vi "LIN Send Single Message.vi"(0 "NAD":u8 format="%.0x", 1 "LIN Device":T1={"Master Frame(3C)"="MasterReq\nSPA3414_ConfigurationsCMAGeely_CEMCALYPSOSDB34XX0Cfg_LIN3_190709_", "Slave Frame(3D)"="SlaveResp\nSPA3414_ConfigurationsCMAGeely_CEMCALYPSOSDB34XX0Cfg_LIN3_190709_", "Request Schedule"="CEMLIN3DiagRequestSchedule\nSPA3414_ConfigurationsCMAGeely_CEMCALYPSOSDB34XX0Cfg_LIN3_190709_", "Response Schedule"="CEMLIN3DiagResponseSchedule\nSPA3414_ConfigurationsCMAGeely_CEMCALYPSOSDB34XX0Cfg_LIN3_190709_", "Frame Write SCU"="", "Frame Read SCU"="", "LIN Name"=""}, 5 "Msg Wait T":u32=3000, 7 "Retries":i32, 9 "FrameCount":i32=1, 11 "error in (no error)":errorcluster, 12 "Need REQ":bool=TRUE, 13 "Tx Msg":u8[][](array[numeric]) format="%.0x") -> (3 "size":i32, 4 "Rx Msg":u8[](array[numeric]) format="%.0x", 6 "TxRx Data":string[][](array[string]), 8 "Response Good?":bool, 10 "spreadsheet String":string, 15 "error OUT":errorcluster caption="error in (no error)")   [LabVIEW 2018]
uses:
  LIN Device.ctl
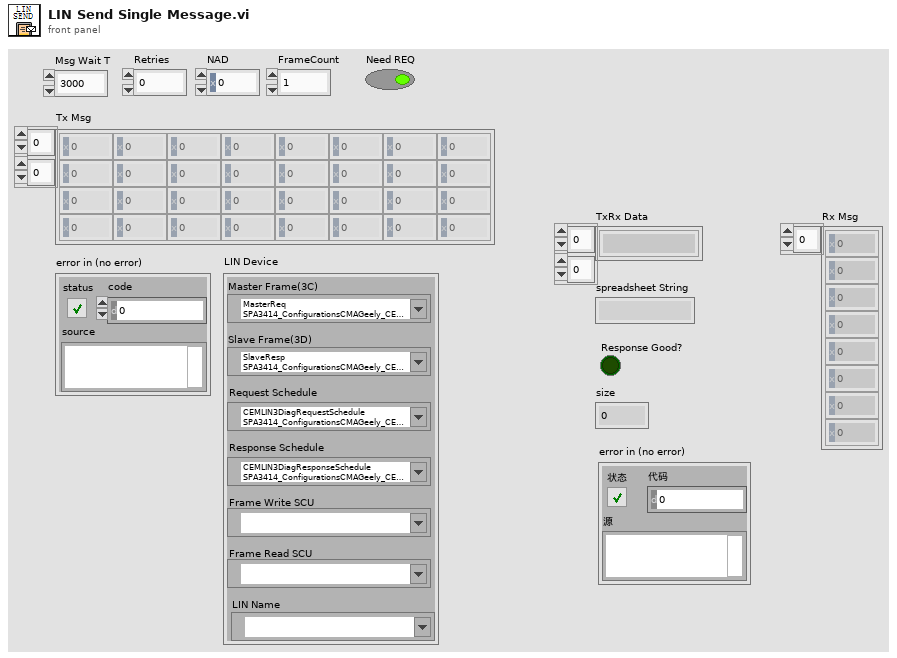
[diagram p1: front panel]
types:
  T1 = typedef "LIN Device.ctl" = cluster{"Master Frame(3C)":refnum<k21>, "Slave Frame(3D)":refnum<k21>, "Request Schedule":refnum<k21>, "Response Schedule":refnum<k21>, "Frame Write SCU":refnum<k21>, "Frame Read SCU":refnum<k21>, "LIN Name":refnum<k21>}
  T2 = cluster{"Tx Msg":u8[][], "NAD":u8, "Retry Counter":i32, "Rx Msg":u8[], "FrameCount":i32, "FF":u8[], "Response Good?":bool, "TxRx Data":string[][], "Message Start Timer":u32, "LIN Device":T1, "element":string[]}
  T3 = typedef "XNET Frame LIN.ctl" = cluster{"timestamp":timestamp, "payload":u8[], "identifier":u32, "type":T4, "event ID":u8, "event slot?":bool, "echo?":bool}
  T4 = typedef "XNET Frame Type LIN.ctl" = u8
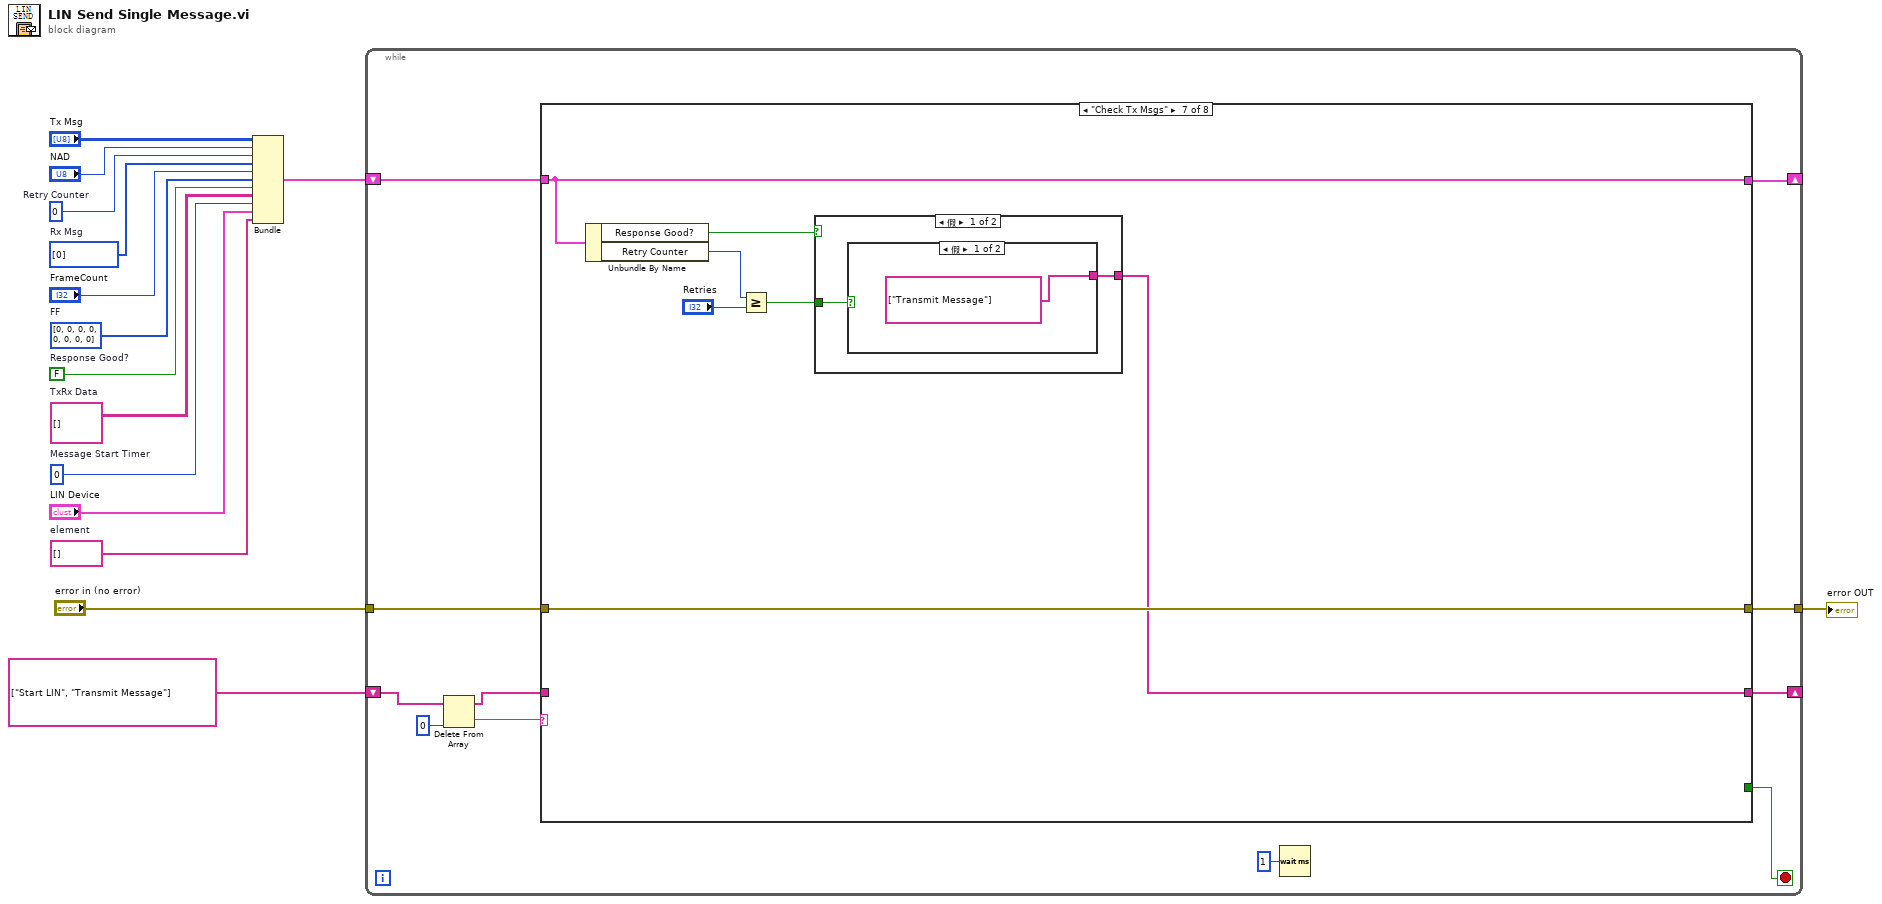
[diagram p0: block diagram]
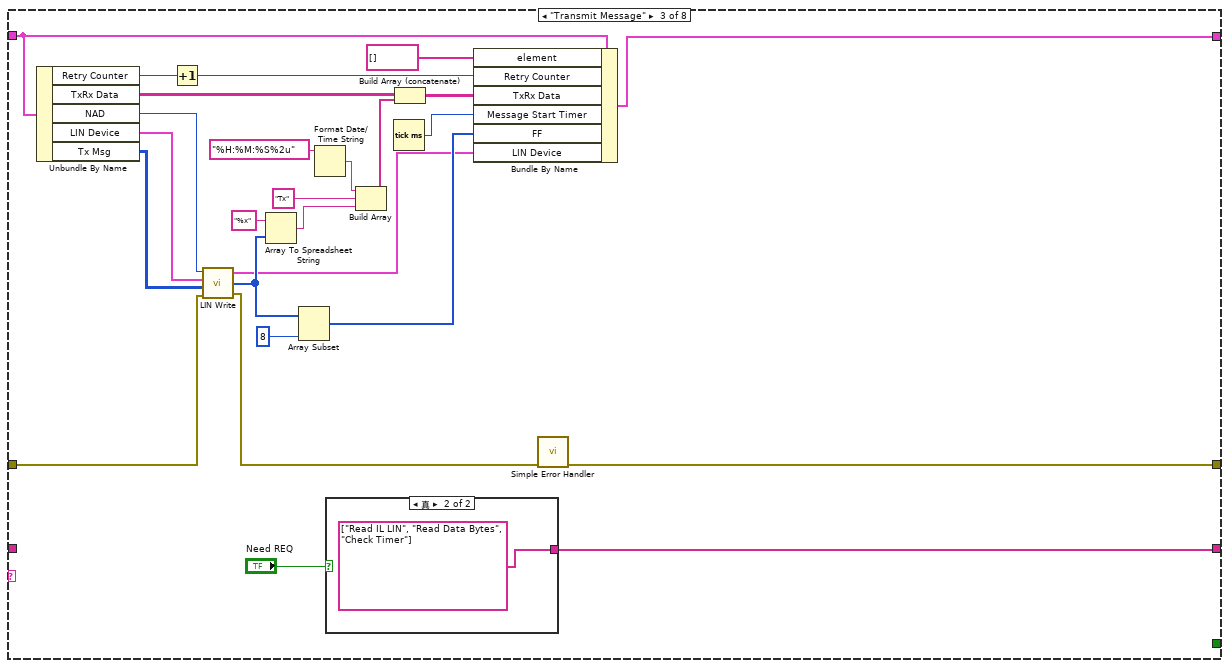
[diagram p4: hidden frame]
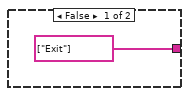
[diagram p5: hidden frame]
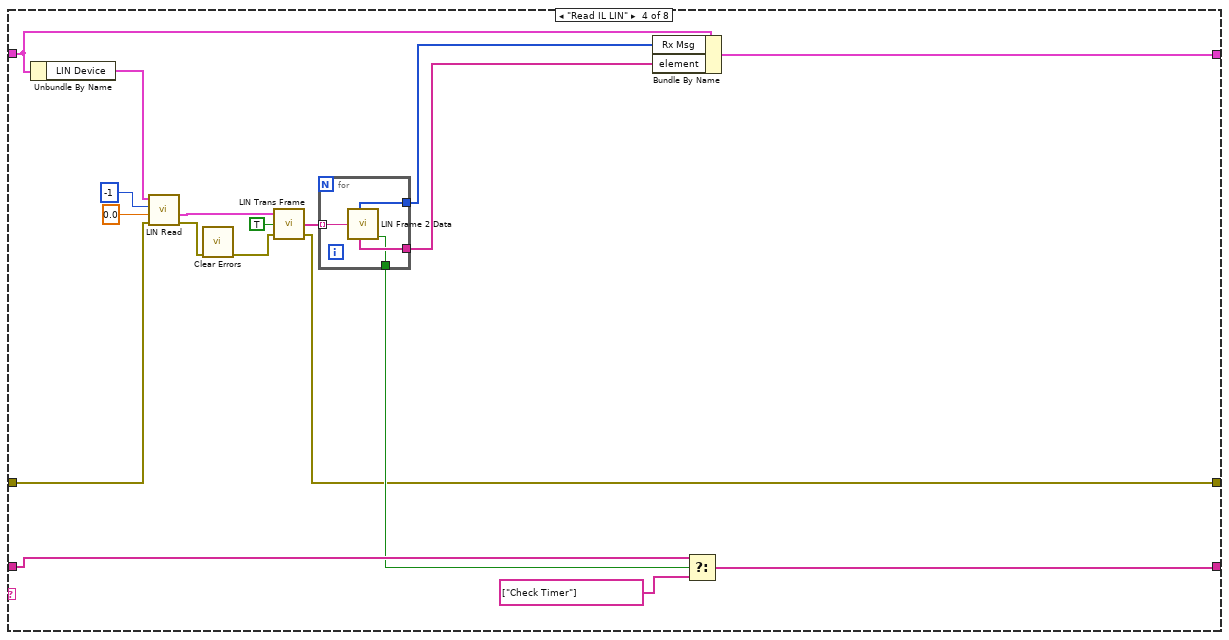
[diagram p6: hidden frame]
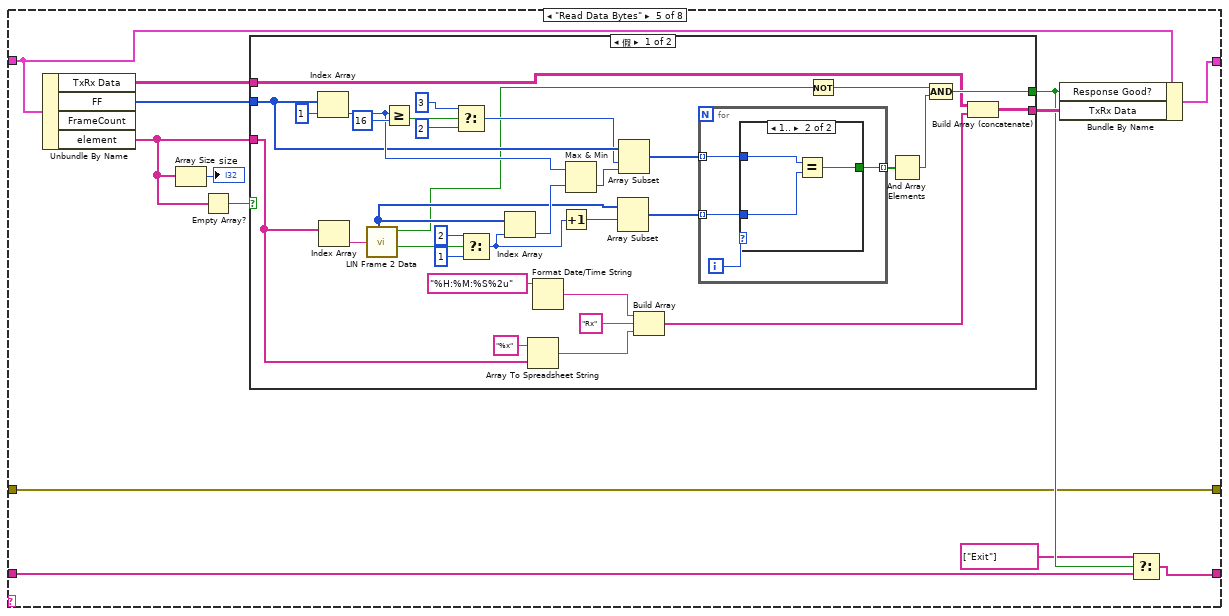
[diagram p7: hidden frame]
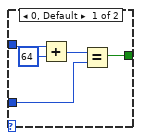
[diagram p8: hidden frame]
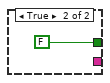
[diagram p9: hidden frame]
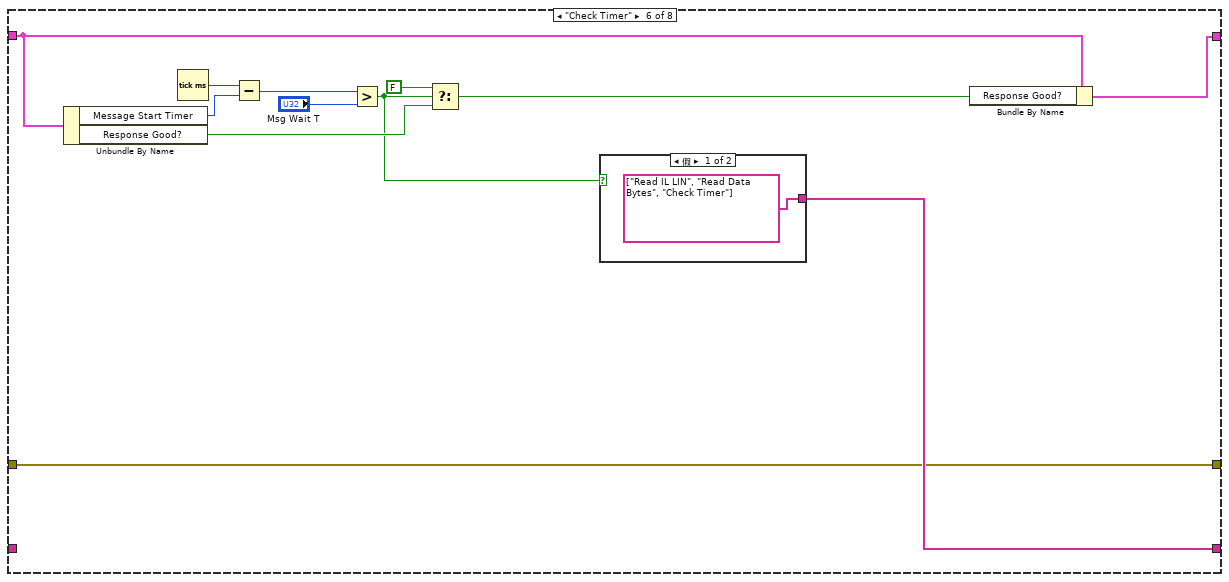
[diagram p10: hidden frame]
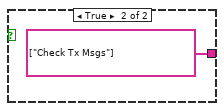
[diagram p11: hidden frame]
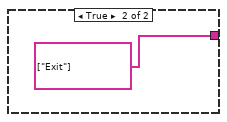
[diagram p12: hidden frame]
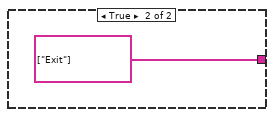
[diagram p13: hidden frame]
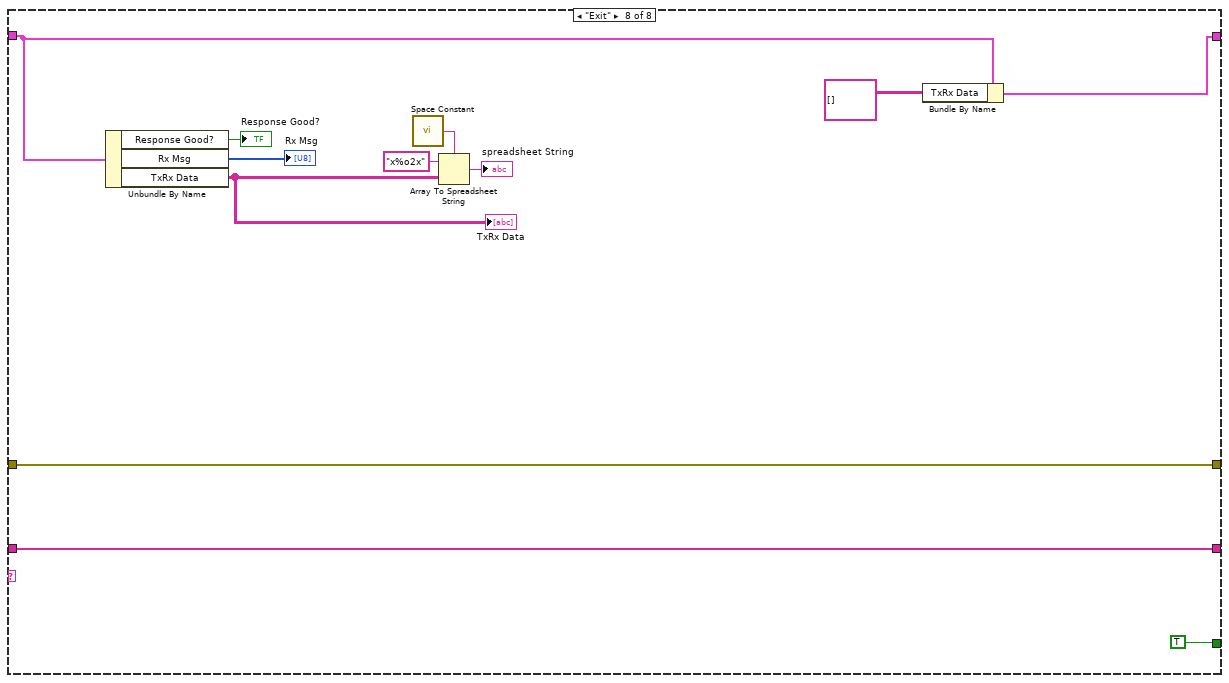
[diagram p14: hidden frame]
diagram:
  w1 = string[] []  # element
  w7 = u32 0  # Message Start Timer
  w8 = string[][] []  # TxRx Data
  w9 = FALSE  # Response Good?
  w10 = u8[] [0, 0, 0, 0, 0, 0, 0, 0]  # FF
  w12 = u8[] [0]  # Rx Msg
  w13 = 0  # Retry Counter
  n1 = Bundle("Tx Msg"="Tx Msg", "NAD"="NAD", "Retry Counter"=w13, "Rx Msg"=w12, "FrameCount"="FrameCount", "FF"=w10, "Response Good?"=w9, "TxRx Data"=w8, "Message Start Timer"=w7, "LIN Device"="LIN Device", "element"=w1) -> (w6:T2)  [unwired: 1 in]
  n2 = while {
    tunnel: "error in (no error)" -> [w23]
    shift-right: [w21] -> _
    shift-left: string[] ["Start LIN", "Transmit Message"] -> [w22]
    shift-right: [w24] -> _
    shift-left: w6 -> [w25]
    tunnel: [w20] -> w3
    stop <- w18 stop-if-true
    n3 = Delete From Array(array=w22, index=0 ("索引")) -> (deleted portion=w26:string, array with subset deleted=w16:string[])  [unwired: 1 in]
    n4 = case shown="\"Check Tx Msgs\"" w26 {
      tunnel: w25 -> [w29 w32 w46 w69 w94 w147 w156 w171]
      tunnel: [w29 w32 w36 w68 w92 w146 w156 w170] -> w24
      tunnel: w23 -> [w28 w30 w49 w75 w83 w142 w162 w172]
      tunnel: w16 -> [w27 w31 _ w64 w84 _ _ w173]
      tunnel: [w27 w31 w35 w65 w87 w143 w157 w173] -> w21
      tunnel: [w28 w30 w38 w61 w83 w142 w162 w172] -> w20
      tunnel: [_ _ _ _ _ _ _ TRUE] -> w18
      frame "Error", Default {
      }
      frame "Start LIN" {
      }
      frame "Transmit Message" {
        n5 = Unbundle By Name(w46) -> ("Retry Counter"=w55:i32, "TxRx Data"=w48:string[][], "NAD"=w58:u8, "LIN Device"=w57:T1, "Tx Msg"=w56:u8[][])
        n6 = Increment(x=w55) -> (x+1=w40:i32)
        n7 = call "LIN Write.vi"("Error IN"=w49, "Tx Msg"=w56, "LIN Device IN"=w57, "NAD"=w58) -> ("error out"=w37:errorcluster, "Array"=w43:u8[], "LIN Device OUT"=w41:T1)
        n8 = Array To Spreadsheet String(array=w43, 3:"%x" ("格式字符串")) -> (spreadsheet string=w50:string)  [unwired: 1 in]
        n9 = Array Subset(array=w43, length=8 ("索引")) -> (w42:u8[])  [unwired: 1 in]
        n10 = Format Date/Time String(time format string (%c)="%H:%M:%S%2u") -> (date/time string=w53:string)  [unwired: 2 in]
        n11 = case shown="真" "Need REQ" {
          tunnel: [string[] ["Exit"] string[] ["Read IL LIN", "Read Data Bytes", "Check Timer"]] -> w35
          frame False {
          }
          frame True {
          }
        }
        n12 = Build Array(w53, "Tx" ("元素"), w50) -> (w47:string[])
        n13 = Tick Count (ms)() -> (millisecond timer value=w44:u32)
        n14 = Build Array (concatenate)(w48, w47) -> (w45:string[][])
        n15 = Bundle By Name(cluster=w46, "element"=string[] [], "Retry Counter"=w40, "TxRx Data"=w45, "Message Start Timer"=w44, "FF"=w42, "LIN Device"=w41) -> (w36:T2)
        n16 = call <vilib>:"Simple Error Handler.vi"("error in (no error)"=w37) -> ("error out"=w38:errorcluster)  [unwired: 4 in, 4 out]
      }
      frame "Read IL LIN" {
        n17 = Unbundle By Name(w69) -> ("LIN Device"=w78:T1)
        n18 = call "LIN Read.vi"("error in (no error)"=w75, "timeout (0)"=0.0, "number to read (-1)"=-1, "LIN Device IN"=w78) -> ("error out"=w74:errorcluster, "data"=w73:T3[])  [unwired: 2 out]
        n19 = call <vilib>:"Clear Errors.vi"("error in (no error)"=w74) -> ("error out"=w71:errorcluster)  [unwired: 5 in, 1 out]
        n20 = call "LIN Trans Frame.vi"("error in (no error)"=w71, "Hex and Dec"=TRUE, "data IN"=w73) -> ("error OUT"=w61:errorcluster, "Data Byte"=w70:string[])  [unwired: 1 out]
        n21 = for {
          tunnel: w70 -> [w82] mode=indexing
          tunnel: [w81] -> w67
          tunnel: [w80] -> w66
          tunnel: [w79] -> w62
          n22 = call "LIN Frame 2 Data.vi"("Frame"=w82) -> ("Array OUT"=w81:u8[], "Element"=w80:string[], "Finish?"=w79:bool)  [unwired: 2 in, 3 out]
        }
        n23 = Bundle By Name(cluster=w69, "Rx Msg"=w67, "element"=w66) -> (w68:T2)
        n24 = Select(t=w64, s=w62, f=string[] ["Check Timer"]) -> (s? t:f=w65:string[])
      }
      frame "Read Data Bytes" {
        n25 = Unbundle By Name(w94) -> ("TxRx Data"=w95:string[][], "FF"=w90:u8[], "element"=w88:string[])  [unwired: 1 out]
        n26 = Array Size(array=w88) -> (size(s)=→"size":i32)
        n27 = Empty Array?(array=w88) -> (empty?=w89:bool)
        n28 = case shown="假" w89 {
          tunnel: w95 -> [w98 _]
          tunnel: [w105 FALSE] -> w86
          tunnel: [w96 _] -> w93
          tunnel: w90 -> [w117 _]
          tunnel: w88 -> [w103 _]
          frame False {
            n29 = Index Array(array=w117, index=1 ("索引")) -> (element=w118:u8)
            n30 = Index Array(array=w103) -> (element=w128:string)  [unwired: 1 in]
            n31 = call "LIN Frame 2 Data.vi"("Frame"=w128) -> ("Array OUT"=w113:u8[], "Error?"=w107:bool, "MulFrame"=w122:bool)  [unwired: 2 in, 3 out]
            n32 = Greater Or Equal?(x=w118, y=u8 16) -> (x >= y?=w125:bool)
            n33 = Select(t=u8 3 ("y"), s=w125, f=u8 2 ("y")) -> (s? t:f=w116:u8)
            n34 = Select(t=u8 2 ("y"), s=w122, f=u8 1 ("y")) -> (s? t:f=w112:u8)
            n35 = Index Array(array=w113, index=w112) -> (element=w119:u8)
            n36 = Array To Spreadsheet String(array=w103, 3:"%x" ("格式字符串")) -> (spreadsheet string=w99:string)  [unwired: 1 in]
            n37 = Format Date/Time String(time format string (%c)="%H:%M:%S%2u") -> (date/time string=w101:string)  [unwired: 2 in]
            n38 = Increment(x=w112) -> (x+1=w111:u8)
            n39 = Max & Min(x=w118, y=w119) -> (min(x,y)=w115:u8)  [unwired: 1 out]
            n40 = Array Subset(array=w113, index=w111) -> (w110:u8[])  [unwired: 1 in]
            n41 = Array Subset(array=w117, index=w116, length=w115) -> (w114:u8[])
            n42 = Build Array(w101, "Rx" ("格式字符串"), w99) -> (w97:string[])
            n43 = for {
              tunnel: w114 -> [w131] mode=indexing
              tunnel: w110 -> [w130] mode=indexing
              tunnel: [w129] -> w109 mode=indexing
              i -> [w132]
              n44 = case shown="1.." w132 {
                tunnel: w131 -> [w137 w139]
                tunnel: w130 -> [w134 w138]
                tunnel: [w133 w140] -> w129
                frame 0, Default {
                  n45 = Add(x=w137, y=u8 64) -> (x+y=w135:u8)
                  n46 = Equal?(x=w135, y=w134) -> (x = y?=w133:bool)
                }
                frame 1.. {
                  n47 = Equal?(x=w139, y=w138) -> (x = y?=w140:bool)
                }
              }
            }
            n48 = Not(x=w107) -> (.not. x?=w106:bool)
            n49 = And Array Elements(Boolean array=w109) -> (logical AND=w108:bool)
            n50 = Compound Arithmetic op=AND ("复合运算")(w106, w108) -> (w105:bool)
            n51 = Build Array (concatenate)(w98, w97) -> (w96:string[][])
          }
          frame True {
          }
        }
        n52 = Bundle By Name(cluster=w94, "Response Good?"=w86, "TxRx Data"=w93) -> (w92:T2)
        n53 = Select(t=string[] ["Exit"], s=w86, f=w84) -> (s? t:f=w87:string[])
      }
      frame "Check Timer" {
        n54 = Unbundle By Name(w147) -> ("Message Start Timer"=w152:u32, "Response Good?"=w148:bool)
        n55 = Tick Count (ms)() -> (millisecond timer value=w153:u32)
        n56 = Subtract(x=w153, y=w152) -> (x-y=w151:u32)
        n57 = Greater?(x=w151, y="Msg Wait T") -> (0:w144:bool)
        n58 = Select(t=FALSE, s=w144, f=w148) -> (s? t:f=w145:bool)
        n59 = case shown="假" w144 {
          tunnel: [string[] ["Read IL LIN", "Read Data Bytes", "Check Timer"] string[] ["Check Tx Msgs"]] -> w143
          frame False {
          }
          frame True {
          }
        }
        n60 = Bundle By Name(cluster=w147, "Response Good?"=w145) -> (w146:T2)
      }
      frame "Check Tx Msgs" {
        n61 = Unbundle By Name(w156) -> ("Response Good?"=w161:bool, "Retry Counter"=w160:i32)
        n62 = Greater Or Equal?(x=w160, y="Retries") -> (x >= y?=w158:bool)
        n63 = case shown="假" w161 {
          tunnel: w158 -> [w164 _]
          tunnel: [w163 string[] ["Exit"]] -> w157
          frame False {
            n64 = case shown="假" w164 {
              tunnel: [string[] ["Transmit Message"] string[] ["Exit"]] -> w163
              frame False {
              }
              frame True {
              }
            }
          }
          frame True {
          }
        }
      }
      frame "Exit" {
        n65 = Unbundle By Name(w171) -> ("Response Good?"=→"Response Good?":bool, "Rx Msg"=→"Rx Msg":u8[], "TxRx Data"=w177:string[][])
        "TxRx Data" <- w177
        n66 = call <vilib>:"Space Constant.vi"() -> ("String"=w175:string)
        n67 = Array To Spreadsheet String(delimiter (Tab)=w175, array=w177, 3:"x%o2x" ("格式字符串")) -> (spreadsheet string=→"spreadsheet String":string)
        n68 = Bundle By Name(cluster=w171, "TxRx Data"=string[][] []) -> (w170:T2)
      }
    }
    n69 = Wait (ms)(milliseconds to wait=u32 1 ("等待时间（毫秒）")) -> ()  [unwired: 1 out]
  }
  "error OUT" <- w3
